vi "Calculando_valores_osciloscopio.vi"() -> ()   [LabVIEW 2014]
uses:
  <vilib>/Utility/file.llb/Read From Spreadsheet File (DBL).vi
  <vilib>/Utility/file.llb/Write To Spreadsheet File (DBL).vi
panel:
  out "Espectro Voltaje":T1(graph)
  in  "file path (dialog if empty) 2":path
  out "appended array":dbl[][](array[numeric])
  in  "file path (dialog if empty)":path=path "I:/Mediciones/bombillo100004.csv"
  out "output cluster":T2 {"Frecuencia" format="%.3g"; "THD V" format="%.3g"; "THD I" format="%.3g"; "FDP" format="%.3g"; "Potencia Activa" format="%.3g"; "Potencia Reactiva" format="%.3g"; "Potencia Aparente" format="%.3g"; "Desfasaje (FDP)" format="%.3g"; "Desfasaje (TM)" format="%.3g"; "Flujo" format="%.3g"; "Vrms" format="%.3g"; "Irms" format="%.3g"; "Energia" format="%.3g"}
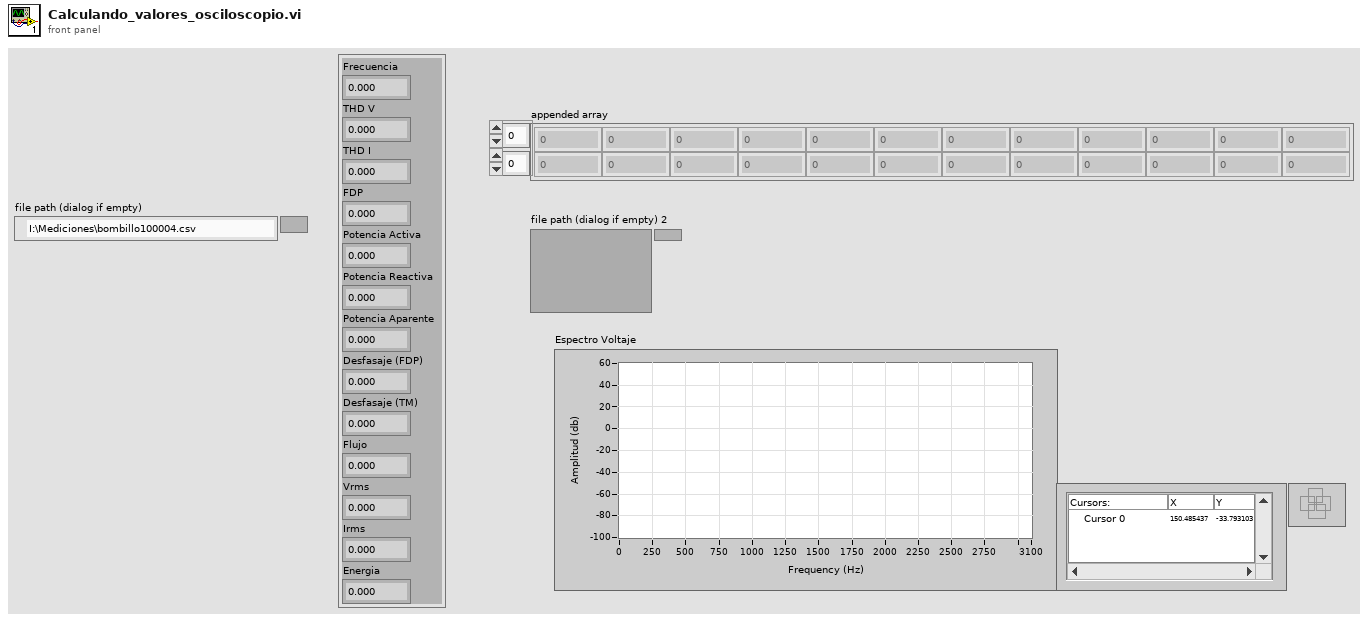
[diagram p1: front panel]
types:
  T1 = cluster{"f0":dbl, "df":dbl, "dB Spectrum (Hann)":dbl[]}
  T2 = cluster{"Frecuencia":dbl, "THD V":dbl, "THD I":dbl, "FDP":dbl, "Potencia Activa":dbl, "Potencia Reactiva":dbl, "Potencia Aparente":dbl, "Desfasaje (FDP)":dbl, "Desfasaje (TM)":dbl, "Flujo":dbl, "Vrms":dbl, "Irms":dbl, "Energia":dbl}
  T3 = cluster{"components level":dbl[], "exported spectrum (dB)":cluster{"f0":dbl, "df":dbl, "dB Spectrum (Hann)":dbl[]}, "Waveform":waveform(dbl), "Power Spectrum (V^2 rms)":dbl[]}
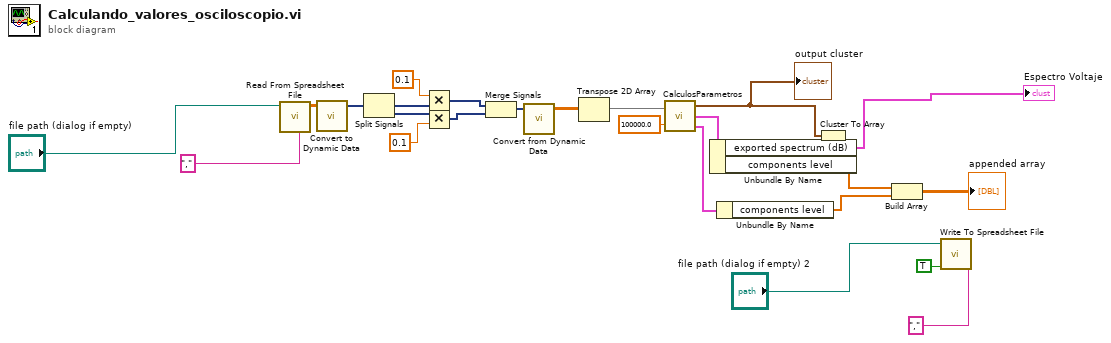
[diagram p0: block diagram]
diagram:
  n1 = call-poly <vilib>:"Read From Spreadsheet File.vi"("delimiter (\\t)"="," ("delimiter (\\t)"), "file path (dialog if empty)"="file path (dialog if empty)") -> ("all rows"=w22:dbl[][])  [unwired: 5 in, 4 out]
  n2 = call "Convert to Dynamic Data"("2D Array"=w22) -> ("Dynamic Data Type"=w21:dynamicdata)  [unwired: 3 in]
  n3 = Split Signals(w21) -> (w14:dynamicdata, w13:dynamicdata)  [unwired: 3 in, 1 out]
  n4 = Multiply(x=0.1, y=w14) -> (x*y=w16:dynamicdata)
  n5 = Multiply(x=w13, y=0.1 ("x")) -> (x*y=w12:dynamicdata)
  n6 = Merge Signals(w16, w12) -> (w20:dynamicdata)
  n7 = call "Convert from Dynamic Data"("Dynamic Data Type"=w20) -> ("Array"=w18:dbl[][])  [unwired: 3 in]
  n8 = Transpose 2D Array(2D array=w18) -> (transposed array=w17:dbl[][])
  n9 = call "CalculosParametros.vi"("2D Array"=w17, "Frecuencia \nMuestreo"=100000.0 ("Frecuencia \nMuestreo")) -> ("output cluster"=w3:T2, "Voltaje"=w9:T3, "Corriente"=w10:T3)
  "output cluster" <- w3
  n10 = Unbundle By Name(w9) -> ("exported spectrum (dB)"=→"Espectro Voltaje":T1, "components level"=w8:dbl[])
  n11 = Unbundle By Name(w10) -> ("components level"=w7:dbl[])
  n12 = Cluster To Array(cluster=w3) -> ()  [unwired: 1 out]
  n13 = Build Array(w8, w7) -> (→"appended array":dbl[][])
  n14 = call-poly <vilib>:"Write To Spreadsheet File.vi"("delimiter (\\t)"="," ("delimiter (\\t)"), "append to file? (new file:F)"=TRUE, "file path (dialog if empty)"="file path (dialog if empty) 2") -> ()  [unwired: 5 in, 1 out]
